vi "ATS_Device.vi"(7 "BoardToVerify":string, 8 "error in (no error)":errorcluster, 9 "ATS_Check":T1, 10 "DevCtrl":T4, 11 "DeviceIn":i32) -> (0 "error out":errorcluster, 1 "NewData":bool, 2 "Device_Status":cluster{"Arm":bool, "Trigger":bool, "Busy":bool}, 3 "DeviceOut":i32, 4 "Sys_Out":T2={"MS_Mode"=FALSE, "MBoard"=0, "#Board"=1}, 5 "DevInfo":T3={"Handle"=0, "Board"="", "CPLD"="", "MemorySize"=0, "SampleSize"=0, "ID"=0, "High_Memory"=FALSE, "Chan/Board"=2}, 6 "#Sys/Brd":i32)   [LabVIEW 2014]
doc: "_____AlazarTech, Scope_____\n\nControl of the device.\n\nInput:\n\"DeviceCtrl option\"\n-Status: read the status of the Device (Arm, Trigger, Busy)\n-About: display the version of the software on all Device.\n-Arm: arm the Device\n-ForceTrig: force the trigger of the device.\n-Abort: stop any action of the device including trigger and acquisition.\n-Initialize: check for all device, open communication and reset parameters.\n-Info: get the info of the device\n-Close: end communication with all device and clear parameters.\n-Calibrate: start the autocalibration procedure of the device.\n-SetManually: open front panel and set parameters manually.\n\"DeviceIn\" = board to access.\n\"ATS_Check\": option to verify at Initializing state.\n\nOutput:\n\"#Sys/Brd\" = on Initialize indicate the number of System on computer, otherwise it indicate the number of board in System.\n\"DeviceOut\" = Duplicate of DeviceIn\n\"Device_Status\" = status of the board (Arm, Triggered, Busy)"
uses:
  ATS_ctl/Device_Ctrl.ctl
  ATS_ctl/Device_Info.ctl
  ATS_ctl/ATS_Sys_Info.ctl
  ATS_ctl/ATS_Check_Ctrl.ctl
  ATS_ctl/ATS_Global_Ctrl.ctl
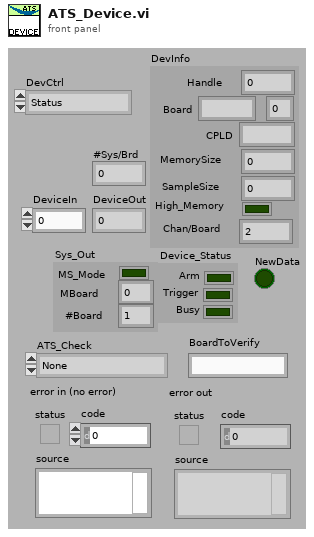
[diagram p1: front panel]
types:
  T1 = typedef "ATS_Check_Ctrl.ctl" = enum16{"None", "NO_ATS9462", "ATS9462_Traditional", "Verify Board", "OnBoard Memory", "Board & Memory", "Master/Slave", "NO Master/Slave"}
  T2 = typedef "ATS_Sys_Info.ctl" = cluster{"MS_Mode":bool, "MBoard":i32, "#Board":i32}
  T3 = typedef "Device_Info.ctl" = cluster{"Handle":u32, "Board":string, "CPLD":string, "MemorySize":u32, "SampleSize":u8, "ID":i32, "High_Memory":bool, "Chan/Board":u8}
  T4 = typedef "Device_Ctrl.ctl" = enum16{"Status", "About", "Arm", "ForceTrig", "Abort", "Initialize", "Init (NoPreset)", "Info", "Close", "Calibrate", "SetManually", "LED_ON", "LED_OFF"}
  T5 = typedef "ATS_Global_Ctrl.ctl" = enum16{"Init_Device", "Clear_ALL", "Set", "Get"}
  T6 = cluster{"Arm":bool, "Trigger":bool, "Busy":bool}[]
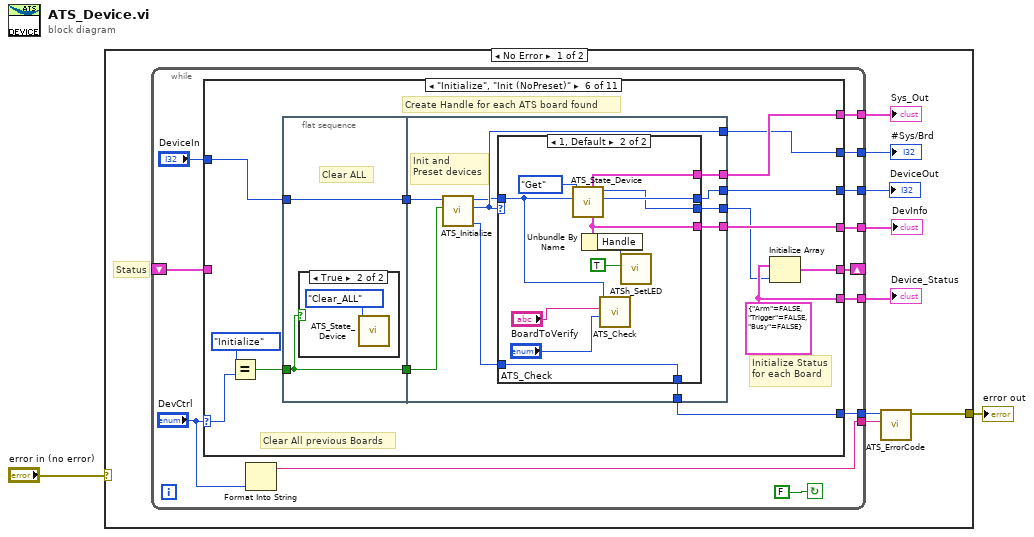
[diagram p0: block diagram]
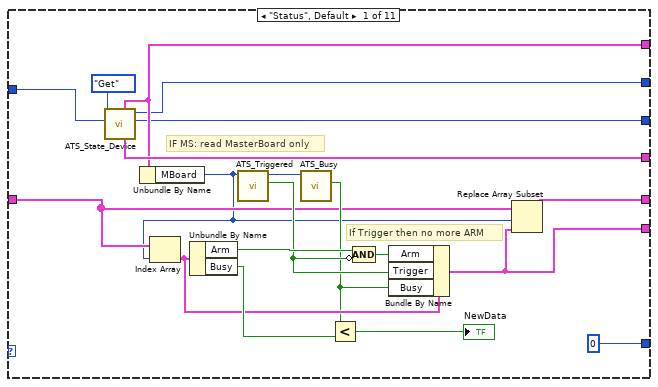
[diagram p2: hidden frame]
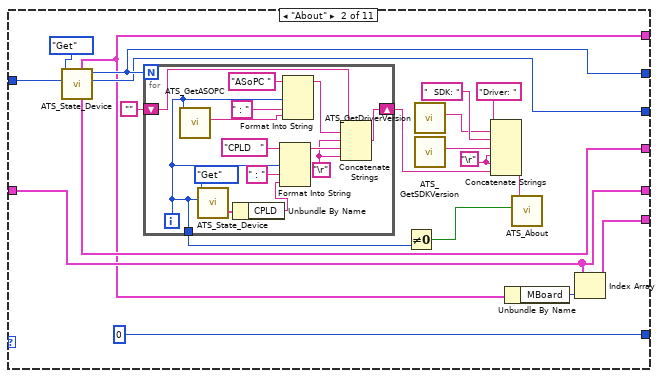
[diagram p3: hidden frame]
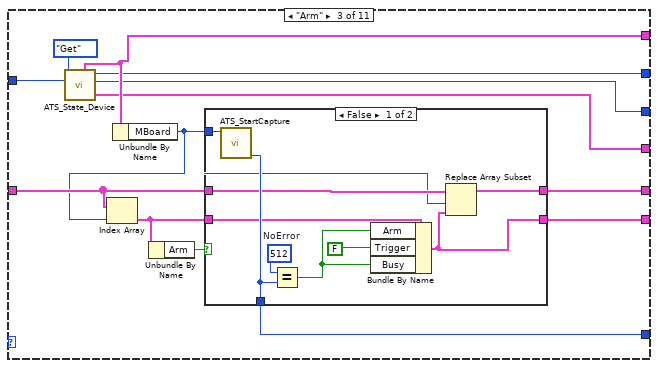
[diagram p4: hidden frame]
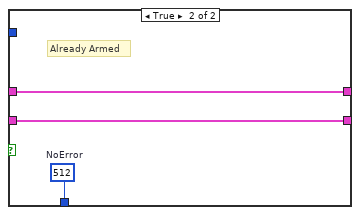
[diagram p5: hidden frame]
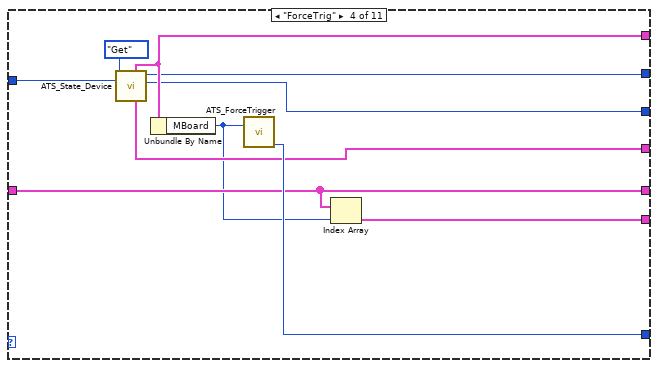
[diagram p6: hidden frame]
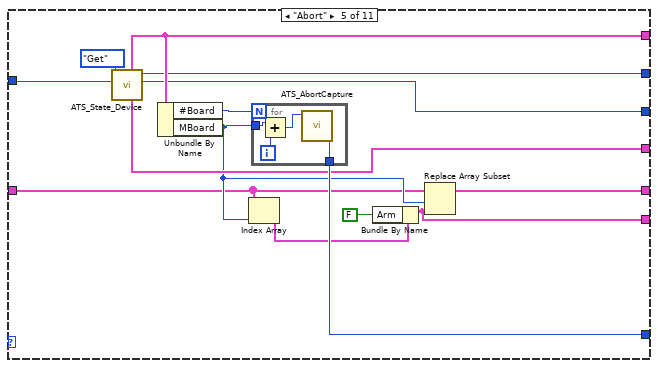
[diagram p7: hidden frame]
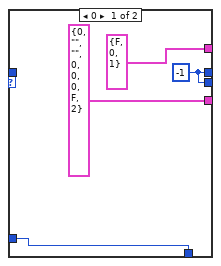
[diagram p9: hidden frame]
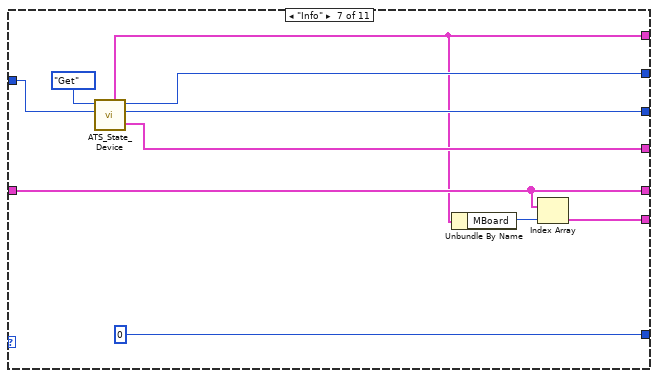
[diagram p10: hidden frame]
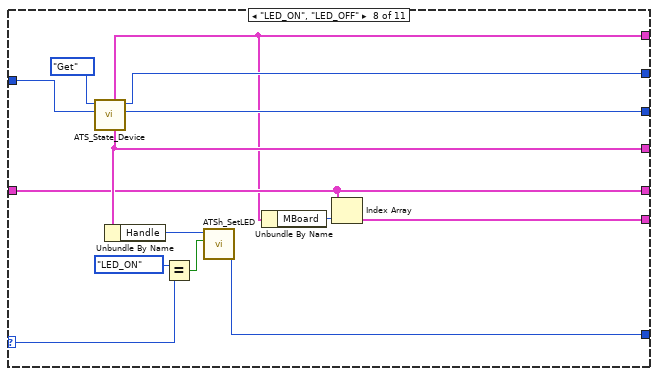
[diagram p11: hidden frame]
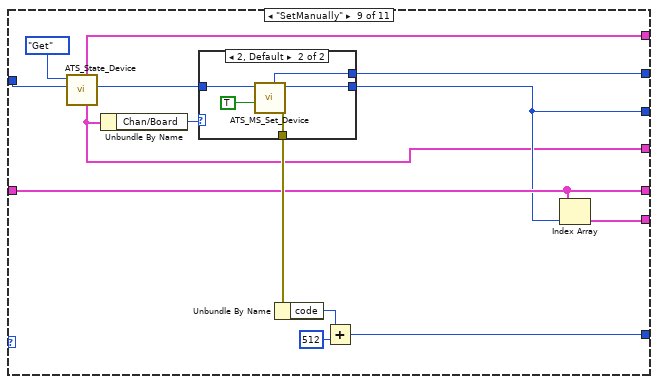
[diagram p12: hidden frame]
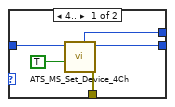
[diagram p13: hidden frame]
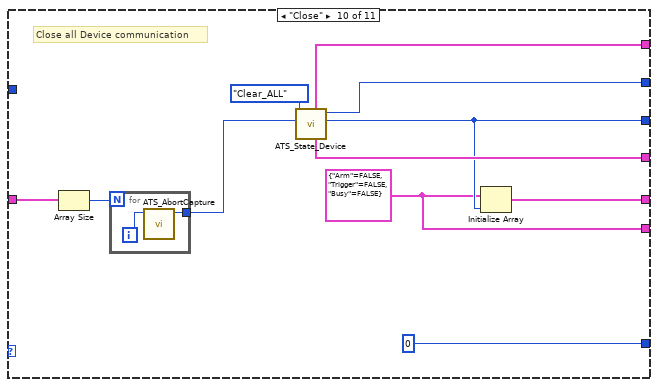
[diagram p14: hidden frame]
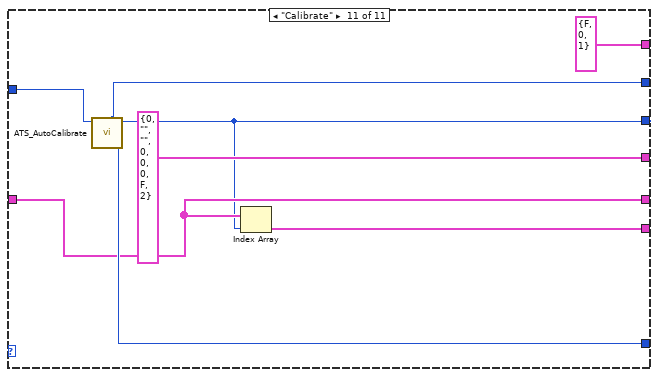
[diagram p15: hidden frame]
diagram:
  n1 = case shown="No Error" "error in (no error)" {
    selector: "error in (no error)" -> [_ w240]
    tunnel: [w9 w240] -> w1
    frame No Error {
      # "Status"
      n2 = while {
        tunnel: [w21] -> w10
        tunnel: [w19] -> w8
        tunnel: [w18] -> w7
        tunnel: [w16] -> w6
        tunnel: [w15] -> w5
        tunnel: [w14] -> w4
        shift-right: [w13] -> _
        shift-left: _ -> [w12]
        tunnel: [w11] -> w3
        stop <- FALSE continue-if-true
        n3 = case shown="\"Initialize\", \"Init (NoPreset)\"" "DevCtrl" {
          selector: "DevCtrl" -> [_ _ _ _ _ w133 _ w188 _ _ _]
          tunnel: [u32 0 u32 0 ("Return Code") w88 w110 w124 w142 u32 0 ("Return Code") w190 w206 u32 0 w239] -> w21
          tunnel: "DeviceIn" -> [w37 w59 w83 w105 w118 w135 w178 w193 w198 _ w238]
          tunnel: [w33 w46 w82 w104 w117 w139 w174 w183 w201 w223 w233] -> w19
          tunnel: [w34 w47 w84 w106 w119 w136 w177 w192 w204 w227 w237] -> w18
          tunnel: [w36 w58 w85 w107 w120 w141 w176 w186 w196 w225 T3 {"Handle"=0, "Board"="", "CPLD"="", "MemorySize"=0, "SampleSize"=0, "ID"=0, "High_Memory"=FALSE, "Chan/Board"=2} ("DevInfo_Out")] -> w15
          tunnel: [w35 w43 w86 w108 w121 w140 w172 w181 w199 w226 T2 {"MS_Mode"=FALSE, "MBoard"=0, "#Board"=1} ("Sys_Out")] -> w14
          tunnel: [w24 w45 w80 w103 w114 w138 w175 w185 w203 w224 w234] -> w13
          tunnel: w12 -> [w26 w45 w79 w103 w111 _ w175 w185 w203 w221 w234]
          tunnel: [w23 w44 w81 w102 w112 w137 w173 w184 w202 w222 w232] -> w11
          frame "Status", Default {
            # "IF MS: read MasterBoard only"
            # "If Trigger then no more ARM"
            n4 = call "ATS_State_Device.vi"("DeviceIn"=w37, "ATS_GBL_Ctrl"=ATS_Global_Ctrl."Get") -> ("DeviceOut"=w33:i32, "#Device"=w34:i32, "DevInfo_Out"=w36:T3, "Sys_Out"=w35:T2)  [unwired: 4 in, 2 out]
            n5 = Unbundle By Name(w35) -> ("MBoard"=w25:i32)
            n6 = Index Array(array=w26, index=w25) -> (element=w30:cluster{"Arm":bool, "Trigger":bool, "Busy":bool})
            n7 = Unbundle By Name(w30) -> ("Arm"=w32:bool, "Busy"=w31:bool)
            n8 = call "ATS_Triggered.vi"("DeviceIn"=w25) -> ("Triggered"=w28:bool, "DeviceOut"=w39:i32)  [unwired: 9 in]
            n9 = call "ATS_Busy.vi"("DeviceIn"=w39) -> ("Busy"=w27:bool)  [unwired: 8 in, 2 out]
            n10 = Less?(x=w27, y=w31) -> (x < y?=→"NewData":bool)
            n11 = Compound Arithmetic op=AND(w32, invert w28) -> (w29:bool)
            n12 = Bundle By Name(cluster=w30, "Arm"=w29, "Trigger"=w28, "Busy"=w27) -> (w23:cluster{"Arm":bool, "Trigger":bool, "Busy":bool})
            n13 = Replace Array Subset(array=w26, new element=w23, index=w25) -> (w24:T6)
          }
          frame "About" {
            w52 = "\r"
            n14 = call "ATS_State_Device.vi"("DeviceIn"=w59, "ATS_GBL_Ctrl"=ATS_Global_Ctrl."Get") -> ("DeviceOut"=w46:i32, "#Device"=w47:i32, "DevInfo_Out"=w58:T3, "Sys_Out"=w43:T2)  [unwired: 4 in, 2 out]
            n15 = for {
              N: w47 -> [_]
              shift-right: [w62] -> w50
              shift-left: "" -> [w67]
              tunnel: [w68] -> w49
              i -> [w68]
              w63 = "\r"
              n16 = call "ATS_GetASOPC.vi"("DeviceIn"=w68) -> ("ASoPC"=w65:string)  [unwired: 7 in, 3 out]
              n17 = call "ATS_State_Device.vi"("DeviceIn"=w68, "ATS_GBL_Ctrl"=ATS_Global_Ctrl."Get") -> ("DevInfo_Out"=w74:T3)  [unwired: 4 in, 5 out]
              n18 = Unbundle By Name(w74) -> ("CPLD"=w71:string)
              n19 = Format Into String(initial string="CPLD   " ("string"), w68, " : " ("string"), w71) -> (resulting string=w64:string)  [unwired: 2 in, 1 out]
              n20 = Format Into String(initial string="ASoPC ", w68, " : " ("string"), w65) -> (resulting string=w70:string)  [unwired: 2 in, 1 out]
              n21 = Concatenate Strings(w67, w70, w63, w64, w63) -> (w62:string)
            }
            n22 = Not Equal To 0?(x=w49) -> (x != 0?=w53:bool)
            n23 = call "ATS_GetDriverVersion.vi"() -> ("Driver_Version"=w55:string)  [unwired: 9 in, 2 out]
            n24 = call "ATS_GetSDKVersion.vi"() -> ("SDK_Version"=w56:string)  [unwired: 9 in, 2 out]
            n25 = Concatenate Strings("Driver: " ("string"), w55, "  SDK: " ("string"), w56, w52, w52, w50) -> (w51:string)
            n26 = Unbundle By Name(w43) -> ("MBoard"=w42:i32)
            n27 = call "ATS_About.vi"("Scrollbar Visible"=w53, "AboutIn"=w51) -> ()  [unwired: 4 in, 2 out]
            n28 = Index Array(array=w45, index=w42) -> (element=w44:cluster{"Arm":bool, "Trigger":bool, "Busy":bool})
          }
          frame "Arm" {
            n29 = call "ATS_State_Device.vi"("DeviceIn"=w83, "ATS_GBL_Ctrl"=ATS_Global_Ctrl."Get") -> ("DeviceOut"=w82:i32, "#Device"=w84:i32, "DevInfo_Out"=w85:T3, "Sys_Out"=w86:T2)  [unwired: 4 in, 2 out]
            n30 = Unbundle By Name(w86) -> ("MBoard"=w78:i32)
            n31 = Index Array(array=w79, index=w78) -> (element=w77:cluster{"Arm":bool, "Trigger":bool, "Busy":bool})
            n32 = Unbundle By Name(w77) -> ("Arm"=w76:bool)
            n33 = case shown="False" w76 {
              tunnel: [w97 w98] -> w88
              tunnel: w77 -> [w95 w99]
              tunnel: [w92 w99] -> w81
              tunnel: [w91 w100] -> w80
              tunnel: w79 -> [w90 w100]
              tunnel: w78 -> [w89 _]
              frame False {
                w96 = u32 512  # NoError
                n34 = call "ATS_StartCapture.vi"("DeviceIn"=w89) -> ("Return Code"=w97:u32)  [unwired: 8 in, 2 out]
                n35 = Equal?(x=w96, y=w97) -> (x = y?=w94:bool)
                n36 = Bundle By Name(cluster=w95, "Arm"=w94, "Trigger"=FALSE, "Busy"=w94) -> (w92:cluster{"Arm":bool, "Trigger":bool, "Busy":bool})
                n37 = Replace Array Subset(array=w90, new element=w92, index=w89) -> (w91:T6)
              }
              frame True {
                w98 = u32 512  # NoError
                # "Already Armed"
              }
            }
          }
          frame "ForceTrig" {
            n38 = call "ATS_State_Device.vi"("DeviceIn"=w105, "ATS_GBL_Ctrl"=ATS_Global_Ctrl."Get") -> ("DeviceOut"=w104:i32, "#Device"=w106:i32, "DevInfo_Out"=w107:T3, "Sys_Out"=w108:T2)  [unwired: 4 in, 2 out]
            n39 = Unbundle By Name(w108) -> ("MBoard"=w101:i32)
            n40 = call "ATS_ForceTrigger.vi"("DeviceIn"=w101) -> ("Return Code"=w110:u32)  [unwired: 8 in, 2 out]
            n41 = Index Array(array=w103, index=w101) -> (element=w102:cluster{"Arm":bool, "Trigger":bool, "Busy":bool})
          }
          frame "Abort" {
            n42 = call "ATS_State_Device.vi"("DeviceIn"=w118, "ATS_GBL_Ctrl"=ATS_Global_Ctrl."Get") -> ("DeviceOut"=w117:i32, "#Device"=w119:i32, "DevInfo_Out"=w120:T3, "Sys_Out"=w121:T2)  [unwired: 4 in, 2 out]
            n43 = Unbundle By Name(w121) -> ("#Board"=w122:i32, "MBoard"=w115:i32)
            n44 = Index Array(array=w111, index=w115) -> (element=w116:cluster{"Arm":bool, "Trigger":bool, "Busy":bool})
            n45 = for {
              N: w122 -> [_]
              tunnel: [w128] -> w124
              tunnel: w115 -> [w125]
              i -> [w127]
              n46 = Add(x=w125, y=w127) -> (x+y=w126:i32)
              n47 = call "ATS_AbortCapture.vi"("DeviceIn"=w126) -> ("Return Code"=w128:u32)  [unwired: 8 in, 2 out]
            }
            n48 = Bundle By Name(cluster=w116, "Arm"=FALSE) -> (w112:cluster{"Arm":bool, "Trigger":bool, "Busy":bool})
            n49 = Replace Array Subset(array=w111, new element=w112, index=w115) -> (w114:T6)
          }
          frame "Initialize", "Init (NoPreset)" {
            w137 = cluster{"Arm":bool, "Trigger":bool, "Busy":bool} {"Arm"=FALSE, "Trigger"=FALSE, "Busy"=FALSE} ("Device_Status")
            # "Initialize Status\nfor each Board"
            # "Clear All previous Boards"
            # "Create Handle for each ATS board found"
            n50 = Equal?(x=Device_Ctrl."Initialize" ("DevCtrl"), y=w133) -> (x = y?=w131:bool)
            n51 = flat-sequence {
              tunnel: w135 -> [w144]
              tunnel: [w144] -> w134
              tunnel: w131 -> [w143]
              tunnel: [w143] -> w130
              tunnel: [w155] -> w142
              tunnel: [w154] -> w141
              tunnel: [w153] -> w140
              tunnel: [w147] -> w139
              tunnel: [w152] -> w136
              tunnel: w134 -> [w151]
              tunnel: w130 -> [w148]
              tunnel: [w146] -> w129
              frame #0 {
                # "Clear ALL"
                n52 = case shown="True" w143 {
                  frame False {
                  }
                  frame True {
                    n53 = call "ATS_State_Device.vi"("ATS_GBL_Ctrl"=ATS_Global_Ctrl."Clear_ALL") -> ()  [unwired: 5 in, 6 out]
                  }
                }
              }
              frame #1 {
                # "Init and\nPreset devices"
                n54 = call "ATS_Initialize.vi"("PreSet_Device"=w148, "Device"=w151) -> ("Code"=w149:i32, "#System"=w152:i32, "DeviceOut"=w150:i32)  [unwired: 7 in]
                n55 = case shown="1, Default" w152 {
                  tunnel: [w157 w164] -> w155
                  tunnel: [T3 {"Handle"=0, "Board"="", "CPLD"="", "MemorySize"=0, "SampleSize"=0, "ID"=0, "High_Memory"=FALSE, "Chan/Board"=2} ("DevInfo_Out") w168] -> w154
                  tunnel: w150 -> [_ w162]
                  tunnel: [T2 {"MS_Mode"=FALSE, "MBoard"=0, "#Board"=1} ("Sys_Out") w166] -> w153
                  tunnel: [w156 w165] -> w147
                  tunnel: w149 -> [w157 w164]
                  tunnel: [w156 w163] -> w146
                  frame 0 {
                    w156 = -1 ("#Device")
                  }
                  frame 1, Default {
                    n56 = call "ATS_State_Device.vi"("DeviceIn"=w162, "ATS_GBL_Ctrl"=ATS_Global_Ctrl."Get") -> ("DeviceOut"=w165:i32, "#Device"=w163:i32, "DevInfo_Out"=w168:T3, "Sys_Out"=w166:T2)  [unwired: 4 in, 2 out]
                    n57 = Unbundle By Name(w168) -> ("Handle"=w167:u32)
                    n58 = call "ATS_Check.vi"("ATS_Check"="ATS_Check", "BoardToVerify"="BoardToVerify", "Device"=w162) -> ()  [unwired: 7 in, 2 out]
                    n59 = call "ATSh_SetLED.vi"("state"=TRUE, "Handle"=w167) -> ()  [unwired: 5 in, 1 out]
                  }
                }
              }
            }
            n60 = Initialize Array(w137, w129) -> (w138:T6)
          }
          frame "Info" {
            n61 = call "ATS_State_Device.vi"("DeviceIn"=w178, "ATS_GBL_Ctrl"=ATS_Global_Ctrl."Get") -> ("DeviceOut"=w174:i32, "#Device"=w177:i32, "DevInfo_Out"=w176:T3, "Sys_Out"=w172:T2)  [unwired: 4 in, 2 out]
            n62 = Unbundle By Name(w172) -> ("MBoard"=w171:i32)
            n63 = Index Array(array=w175, index=w171) -> (element=w173:cluster{"Arm":bool, "Trigger":bool, "Busy":bool})
          }
          frame "LED_ON", "LED_OFF" {
            n64 = call "ATS_State_Device.vi"("DeviceIn"=w193, "ATS_GBL_Ctrl"=ATS_Global_Ctrl."Get") -> ("DeviceOut"=w183:i32, "#Device"=w192:i32, "DevInfo_Out"=w186:T3, "Sys_Out"=w181:T2)  [unwired: 4 in, 2 out]
            n65 = Unbundle By Name(w186) -> ("Handle"=w191:u32)
            n66 = Equal?(x=Device_Ctrl."LED_ON" ("DevCtrl"), y=w188) -> (x = y?=w187:bool)
            n67 = call "ATSh_SetLED.vi"("state"=w187, "Handle"=w191) -> ("Return_Code"=w190:u32)  [unwired: 5 in]
            n68 = Unbundle By Name(w181) -> ("MBoard"=w182:i32)
            n69 = Index Array(array=w185, index=w182) -> (element=w184:cluster{"Arm":bool, "Trigger":bool, "Busy":bool})
          }
          frame "SetManually" {
            n70 = call "ATS_State_Device.vi"("DeviceIn"=w198, "ATS_GBL_Ctrl"=ATS_Global_Ctrl."Get") -> ("DeviceOut"=w197:i32, "DevInfo_Out"=w196:T3, "Sys_Out"=w199:T2)  [unwired: 4 in, 3 out]
            n71 = Unbundle By Name(w196) -> ("Chan/Board"=w195:u8)
            n72 = case shown="2, Default" w195 {
              tunnel: [w212 w217] -> w208
              tunnel: [w211 w216] -> w204
              tunnel: [w210 w215] -> w201
              tunnel: w197 -> [w209 w214]
              frame 4.. {
                n73 = call "ATS_MS_Set_Device_4Ch.vi"("Set_Manually (F)"=TRUE, "DeviceIn"=w209) -> ("error out"=w212:errorcluster, "DeviceOut"=w210:i32, "#Device"=w211:i32)  [unwired: 4 in, 3 out]
              }
              frame 2, Default {
                n74 = call "ATS_MS_Set_Device.vi"("Set_Manually (F)"=TRUE, "DeviceIn"=w214) -> ("error out"=w217:errorcluster, "DeviceOut"=w215:i32, "#Device"=w216:i32)  [unwired: 4 in, 3 out]
              }
            }
            n75 = Unbundle By Name(w208) -> ("code"=w207:i32)
            n76 = Add(x=w207, y=512) -> (x+y=w206:i32)
            n77 = Index Array(array=w203, index=w201) -> (element=w202:cluster{"Arm":bool, "Trigger":bool, "Busy":bool})
          }
          frame "Close" {
            w222 = cluster{"Arm":bool, "Trigger":bool, "Busy":bool} {"Arm"=FALSE, "Trigger"=FALSE, "Busy"=FALSE} ("Device_Status")
            # "Close all Device communication"
            n78 = Array Size(array=w221) -> (size(s)=w220:i32)
            n79 = for {
              N: w220 -> [_]
              tunnel: [w230] -> w219
              i -> [w231]
              n80 = call "ATS_AbortCapture.vi"("DeviceIn"=w231) -> ("DeviceOut"=w230:i32)  [unwired: 8 in, 2 out]
            }
            n81 = call "ATS_State_Device.vi"("DeviceIn"=w219, "ATS_GBL_Ctrl"=ATS_Global_Ctrl."Clear_ALL") -> ("DeviceOut"=w223:i32, "#Device"=w227:i32, "DevInfo_Out"=w225:T3, "Sys_Out"=w226:T2)  [unwired: 4 in, 2 out]
            n82 = Initialize Array(w222, w223) -> (w224:T6)
          }
          frame "Calibrate" {
            n83 = call "ATS_AutoCalibrate.vi"("DeviceIn"=w238) -> ("Return Code"=w239:u32, "DeviceOut"=w233:i32, "#Device"=w237:i32)  [unwired: 8 in]
            n84 = Index Array(array=w234, index=w233) -> (element=w232:cluster{"Arm":bool, "Trigger":bool, "Busy":bool})
          }
        }
        n85 = Format Into String("DevCtrl") -> (resulting string=w16:string)  [unwired: 3 in, 1 out]
      }
      "DeviceOut" <- w8
      "#Sys/Brd" <- w7
      "Device_Status" <- w3
      "Sys_Out" <- w4
      "DevInfo" <- w5
      n86 = call "ATS_ErrorCode.vi"("Message"=w6, "ErrorCode"=w10) -> ("error out"=w9:errorcluster)  [unwired: 5 in]
    }
    frame Error {
    }
  }
  "error out" <- w1
